vi "ArduinoCom.vi"(10 "write buffer":string="b") -> ()   [LabVIEW 2021]
uses:
  <vilib>/Instr/_visa.llb/VISA Configure Serial Port (Instr).vi
panel:
  in  "termination char\n(0xA = '\\n' = LF)":u8=10 format="%.0x"
  out "return count":u32=1
  out "Serial Settings:Number of Bytes at Serial Port":u32=3
  out "read buffer":string="a\r\n"
  in  "flow control (0:none)":u16(ring) items=["None", "XON/XOFF", "RTS/CTS", "XON/XOFF & RTS/CTS", "DTR/DSR", "XON/XOFF & DTR/DSR"]
  in  "stop bits (10: 1 bit)":u16(ring)=10 items=["1.0"=10, "1.5"=15, "2.0"=20]
  in  "parity (0:none)":enum16{"None", "Odd", "Even", "Mark", "Space"}(ring)
  in  "data bits (8)":u16=8 min=5 max=8 step=1
  in  "baud rate (9600)":u32=9600
  in  "VISA resource name":refnum<visa-resource-name>="COM3"
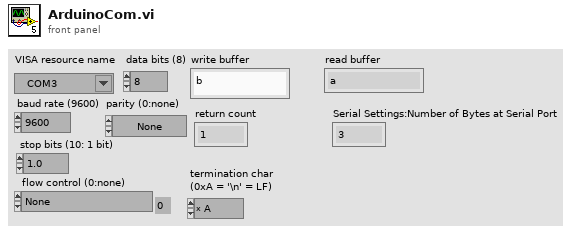
[diagram p1: front panel]
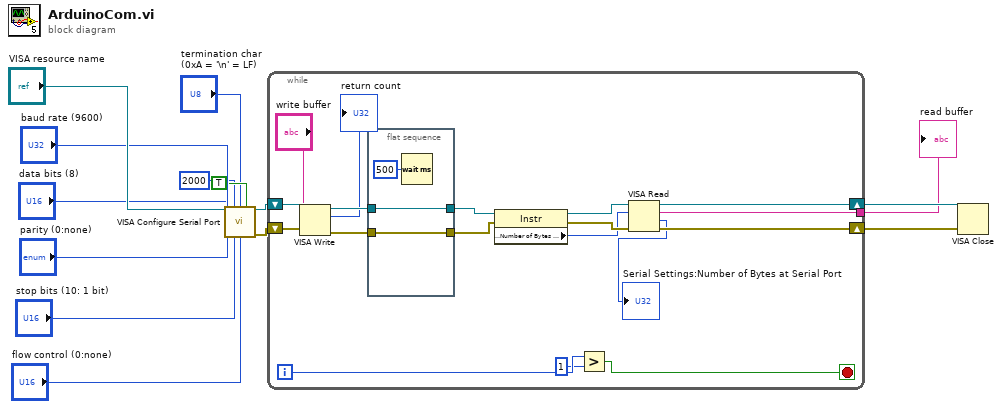
[diagram p0: block diagram]
diagram:
  n1 = call-poly "VISA Configure Serial Port"("VISA resource name"="VISA resource name", "timeout (10sec)"=u32 2000, "termination char\n(0xA = '\\n' = LF)"="termination char\n(0xA = '\\n' = LF)", "Enable Termination\nChar (T)"=TRUE ("Enable Termination\nChar (T)"), "baud rate (9600)"="baud rate (9600)", "data bits (8)"="data bits (8)", "parity (0:none)"="parity (0:none)", "stop bits (10: 1 bit)"="stop bits (10: 1 bit)", "flow control (0:none)"="flow control (0:none)") -> ("VISA resource name out"=w7:refnum<visa-resource-name>, "error out"=w8:errorcluster)  [unwired: 5 in]
  n2 = while {
    tunnel: [w25] -> w4
    shift-right: [w26] -> w5
    shift-left: w8 -> [w32]
    shift-right: [w27] -> w6
    shift-left: w7 -> [w31]
    i -> [w17]
    stop <- w15 stop-if-true
    n3 = VISA Write(VISA resource name=w31, write buffer="write buffer", error in (no error)=w32) -> (VISA resource name out=w29:refnum<visa-resource-name>, return count=→"return count":u32, error out=w28:errorcluster)
    n4 = flat-sequence {
      tunnel: w29 -> [w35]
      tunnel: [w35] -> w24
      tunnel: w28 -> [w34]
      tunnel: [w34] -> w23
      frame #0 {
        n5 = Wait (ms)(milliseconds to wait=u32 500) -> ()  [unwired: 1 out]
      }
    }
    n6 = property class="Instr"(reference=w24, error in=w23) -> (reference out=w22:refnum<visa-resource-name>, error out=w21:errorcluster, "Serial Settings:Number of Bytes at Serial Port"=w20:u32)
    n7 = Greater?(x=w17, y=1) -> (0:w15:bool)
    n8 = VISA Read(VISA resource name=w22, byte count=w20, error in (no error)=w21) -> (VISA resource name out=w27:refnum<visa-resource-name>, read buffer=w25:string, return count=→"Serial Settings:Number of Bytes at Serial Port":u32, error out=w26:errorcluster)
  }
  "read buffer" <- w4
  n9 = VISA Close(VISA resource name=w6, error in (no error)=w5) -> ()  [unwired: 1 out]
